vi "PAN_ConnMngr.vi"(7 "logfile":path, 10 "id":string) -> ()   [LabVIEW 2016]
uses:
  PAN_ConnMngrQStruct.ctl
  public/vis/coms/TCPSERVER/private/vis/PAN_TCPSERVER_ConnectionStruct.ctl
  public/vis/coms/TCPSERVER/private/vis/PAN_TCPSERVER_MngrActionStruct.ctl
panel:
  in  "Cluster":T1
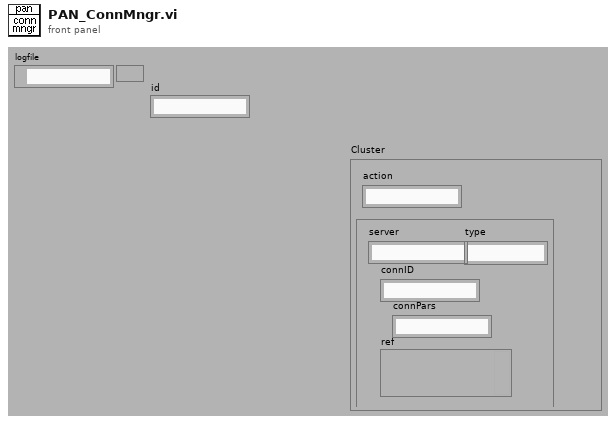
[diagram p1: front panel]
types:
  T1 = typedef "PAN_ConnMngrQStruct.ctl" = cluster{"action":string, "connection":T2}
  T2 = typedef "PAN_TCPSERVER_ConnectionStruct.ctl" = cluster{"ref":variant, "connPars":string, "server":string, "connID":string, "type":string}
  T3 = typedef "PAN_TCPSERVER_MngrActionStruct.ctl" = enum16{"clean", "add", "get all", "find by server", "get servers", "delete", "disconnect", "get connection"}
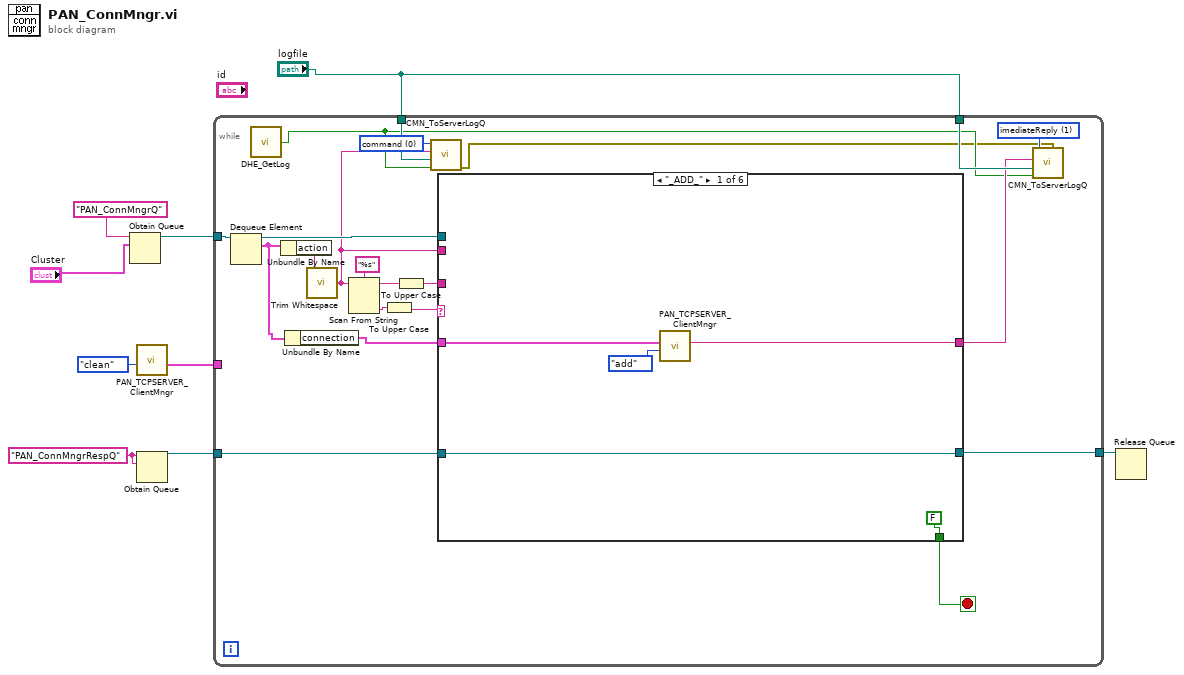
[diagram p0: block diagram]
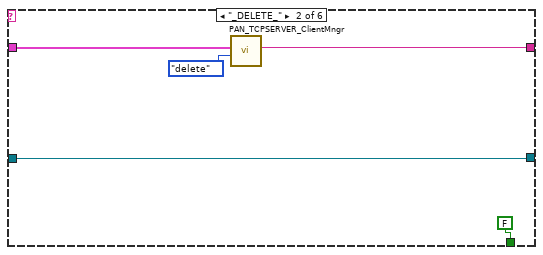
[diagram p2: hidden frame]
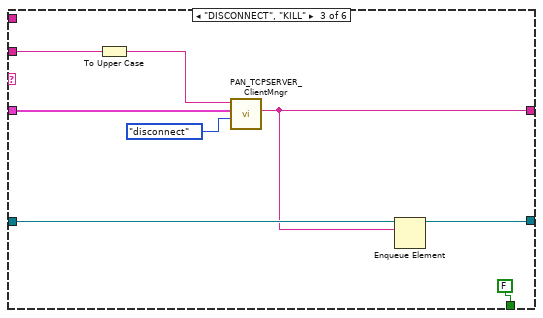
[diagram p3: hidden frame]
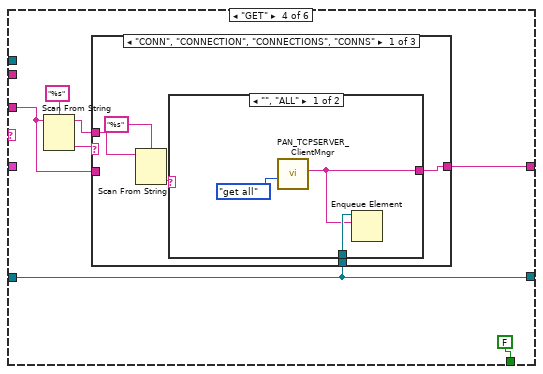
[diagram p4: hidden frame]
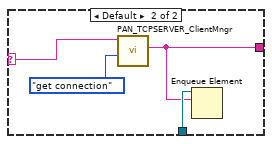
[diagram p5: hidden frame]
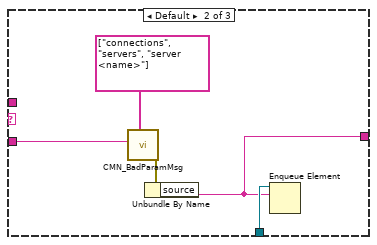
[diagram p6: hidden frame]
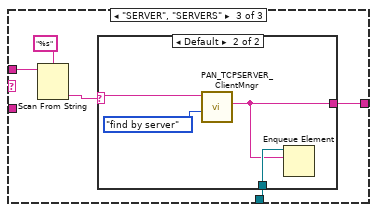
[diagram p7: hidden frame]
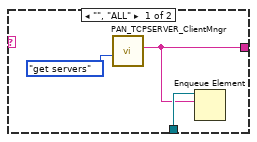
[diagram p8: hidden frame]
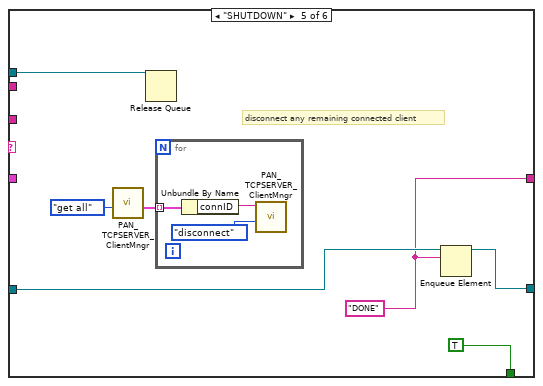
[diagram p9: hidden frame]
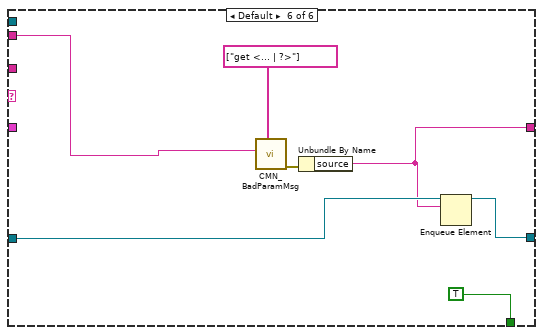
[diagram p10: hidden frame]
diagram:
  w7 = "PAN_ConnMngrRespQ" ("name (unnamed)")
  n1 = Obtain Queue(name (unnamed)="PAN_ConnMngrQ", element data type="Cluster") -> (queue out=w8:refnum<queue>)  [unwired: 3 in, 2 out]
  n2 = call "PAN_TCPSERVER_ClientMngr.vi"("action"=PAN_TCPSERVER_MngrActionStruct."clean") -> ("Clients"=w4:T2[])  [unwired: 2 in, 8 out]
  n3 = Obtain Queue(name (unnamed)=w7, element data type=w7) -> (queue out=w6:refnum<queue>)  [unwired: 3 in, 2 out]
  n4 = while {
    tunnel: w8 -> [w30]
    tunnel: w6 -> [w24]
    tunnel: "logfile" -> [w22]
    tunnel: "logfile" -> [w21]
    tunnel: w4 -> [_]
    tunnel: [w17] -> w3
    stop <- w25 stop-if-true
    w20 = u16 0 items=["command", "imediateReply", "Callback Reply", "Information", "none"] ("type")
    w23 = u16 1 items=["command", "imediateReply", "Callback Reply", "Information"] ("type")
    n5 = Dequeue Element(queue=w30) -> (queue out=w26:refnum<queue>, element=w19:T1)  [unwired: 1 in, 3 out]
    n6 = call "DHE_GetLog.vi"() -> ("DHE_log"=w12:bool)  [unwired: 9 out]
    n7 = Unbundle By Name(w19) -> ("action"=w16:string)
    n8 = Unbundle By Name(w19) -> ("connection"=w18:T2)
    n9 = call <vilib>:"Trim Whitespace.vi"("string"=w16) -> ("trimmed string"=w10:string)  [unwired: 1 in]
    n10 = Scan From String(format string="%s", input string=w10) -> (remaining string=w15:string, output 1=w28:string)  [unwired: 2 in, 3 out]
    n11 = To Upper Case(1:w28) -> (0:w27:string)
    n12 = To Upper Case(1:w15) -> (0:w14:string)
    n13 = call "CMN_ToServerLogQ.vi"("Log"=w12, "file"=w22, "string"=w10, "type"=w20) -> ("error out"=w11:errorcluster)  [unwired: 2 in, 4 out]
    n14 = case shown="\"_ADD_\"" w27 {
      tunnel: w26 -> [_ _ _ _ w91 _]
      tunnel: [FALSE FALSE FALSE FALSE TRUE TRUE] -> w25
      tunnel: w24 -> [w32 w37 w45 w52 w89 w100]
      tunnel: w18 -> [w33 w38 w46 _ _ _]
      tunnel: [w32 w37 w44 w52 w88 w99] -> w17
      tunnel: w10 -> [_ _ _ _ _ w97]
      tunnel: w14 -> [_ _ w43 w50 _ _]
      tunnel: [w31 w36 w41 w49 w87 w95] -> w13
      frame "_ADD_" {
        n15 = call "PAN_TCPSERVER_ClientMngr.vi"("action"=PAN_TCPSERVER_MngrActionStruct."add", "connection"=w33) -> ("resp"=w31:string)  [unwired: 1 in, 8 out]
      }
      frame "_DELETE_" {
        n16 = call "PAN_TCPSERVER_ClientMngr.vi"("action"=PAN_TCPSERVER_MngrActionStruct."delete", "connection"=w38) -> ("resp"=w36:string)  [unwired: 1 in, 8 out]
      }
      frame "DISCONNECT", "KILL" {
        n17 = To Upper Case(1:w43) -> (0:w42:string)
        n18 = call "PAN_TCPSERVER_ClientMngr.vi"("action"=PAN_TCPSERVER_MngrActionStruct."disconnect", "connection"=w46, "args"=w42) -> ("resp"=w41:string)  [unwired: 8 out]
        n19 = Enqueue Element(queue=w45, element=w41) -> (queue out=w44:refnum<queue>)  [unwired: 1 in, 3 out]
      }
      frame "GET" {
        n20 = Scan From String(format string="%s", input string=w50) -> (remaining string=w51:string, output 1=w53:string)  [unwired: 2 in, 3 out]
        n21 = case shown="\"CONN\", \"CONNECTION\", \"CONNECTIONS\", \"CONNS\"" w53 {
          tunnel: w52 -> [w60 w72 w77]
          tunnel: w51 -> [w59 _ w76]
          tunnel: w50 -> [_ w70 _]
          tunnel: [w56 w68 w73] -> w49
          frame "CONN", "CONNECTION", "CONNECTIONS", "CONNS" {
            n22 = Scan From String(format string="%s", input string=w59) -> (output 1=w57:string)  [unwired: 2 in, 4 out]
            n23 = case shown="\"\", \"ALL\"" w57 {
              selector: w57 -> [_ w65]
              tunnel: w60 -> [w63 w67]
              tunnel: [w61 w64] -> w56
              frame "", "ALL" {
                n24 = call "PAN_TCPSERVER_ClientMngr.vi"("action"=PAN_TCPSERVER_MngrActionStruct."get all") -> ("resp"=w61:string)  [unwired: 2 in, 8 out]
                n25 = Enqueue Element(queue=w63, element=w61) -> ()  [unwired: 1 in, 4 out]
              }
              frame Default {
                n26 = call "PAN_TCPSERVER_ClientMngr.vi"("action"=PAN_TCPSERVER_MngrActionStruct."get connection", "args"=w65) -> ("resp"=w64:string)  [unwired: 1 in, 8 out]
                n27 = Enqueue Element(queue=w67, element=w64) -> ()  [unwired: 1 in, 4 out]
              }
            }
          }
          frame Default {
            n28 = call "CMN_BadParamMsg.vi"("valid params"=string[] ["connections", "servers", "server <name>"], "parameter"=w70) -> ("error out"=w71:errorcluster)  [unwired: 2 in, 7 out]
            n29 = Unbundle By Name(w71) -> ("source"=w68:string)
            n30 = Enqueue Element(queue=w72, element=w68) -> ()  [unwired: 1 in, 4 out]
          }
          frame "SERVER", "SERVERS" {
            n31 = Scan From String(format string="%s", input string=w76) -> (output 1=w74:string)  [unwired: 2 in, 4 out]
            n32 = case shown="Default" w74 {
              selector: w74 -> [_ w82]
              tunnel: w77 -> [w79 w83]
              tunnel: [w78 w81] -> w73
              frame "", "ALL" {
                n33 = call "PAN_TCPSERVER_ClientMngr.vi"("action"=PAN_TCPSERVER_MngrActionStruct."get servers") -> ("resp"=w78:string)  [unwired: 2 in, 8 out]
                n34 = Enqueue Element(queue=w79, element=w78) -> ()  [unwired: 1 in, 4 out]
              }
              frame Default {
                n35 = call "PAN_TCPSERVER_ClientMngr.vi"("action"=PAN_TCPSERVER_MngrActionStruct."find by server", "args"=w82) -> ("resp"=w81:string)  [unwired: 1 in, 8 out]
                n36 = Enqueue Element(queue=w83, element=w81) -> ()  [unwired: 1 in, 4 out]
              }
            }
          }
        }
      }
      frame "SHUTDOWN" {
        w87 = "DONE" ("element")
        # "disconnect any remaining connected client"
        n37 = call "PAN_TCPSERVER_ClientMngr.vi"("action"=PAN_TCPSERVER_MngrActionStruct."get all") -> ("Clients"=w85:T2[])  [unwired: 2 in, 8 out]
        n38 = Release Queue(queue=w91) -> ()  [unwired: 1 in, 4 out]
        n39 = for {
          tunnel: w85 -> [w94] mode=indexing
          n40 = Unbundle By Name(w94) -> ("connID"=w93:string)
          n41 = call "PAN_TCPSERVER_ClientMngr.vi"("action"=PAN_TCPSERVER_MngrActionStruct."disconnect", "args"=w93) -> ()  [unwired: 1 in, 9 out]
        }
        n42 = Enqueue Element(queue=w89, element=w87) -> (queue out=w88:refnum<queue>)  [unwired: 1 in, 3 out]
      }
      frame Default {
        n43 = call "CMN_BadParamMsg.vi"("valid params"=string[] ["get <... | ?>"], "parameter"=w97) -> ("error out"=w96:errorcluster)  [unwired: 2 in, 7 out]
        n44 = Unbundle By Name(w96) -> ("source"=w95:string)
        n45 = Enqueue Element(queue=w100, element=w95) -> (queue out=w99:refnum<queue>)  [unwired: 1 in, 3 out]
      }
    }
    n46 = call "CMN_ToServerLogQ.vi"("error in (no error)"=w11, "Log"=w12, "file"=w21, "string"=w13, "type"=w23) -> ()  [unwired: 1 in, 5 out]
  }
  n47 = Release Queue(queue=w3) -> ()  [unwired: 1 in, 4 out]
